vi "DeleteTempFolder.vi"(8 "error in (no error)":errorcluster, 10 "Project":string, 11 "Root":path) -> (0 "error out":errorcluster)   [LabVIEW 2019]
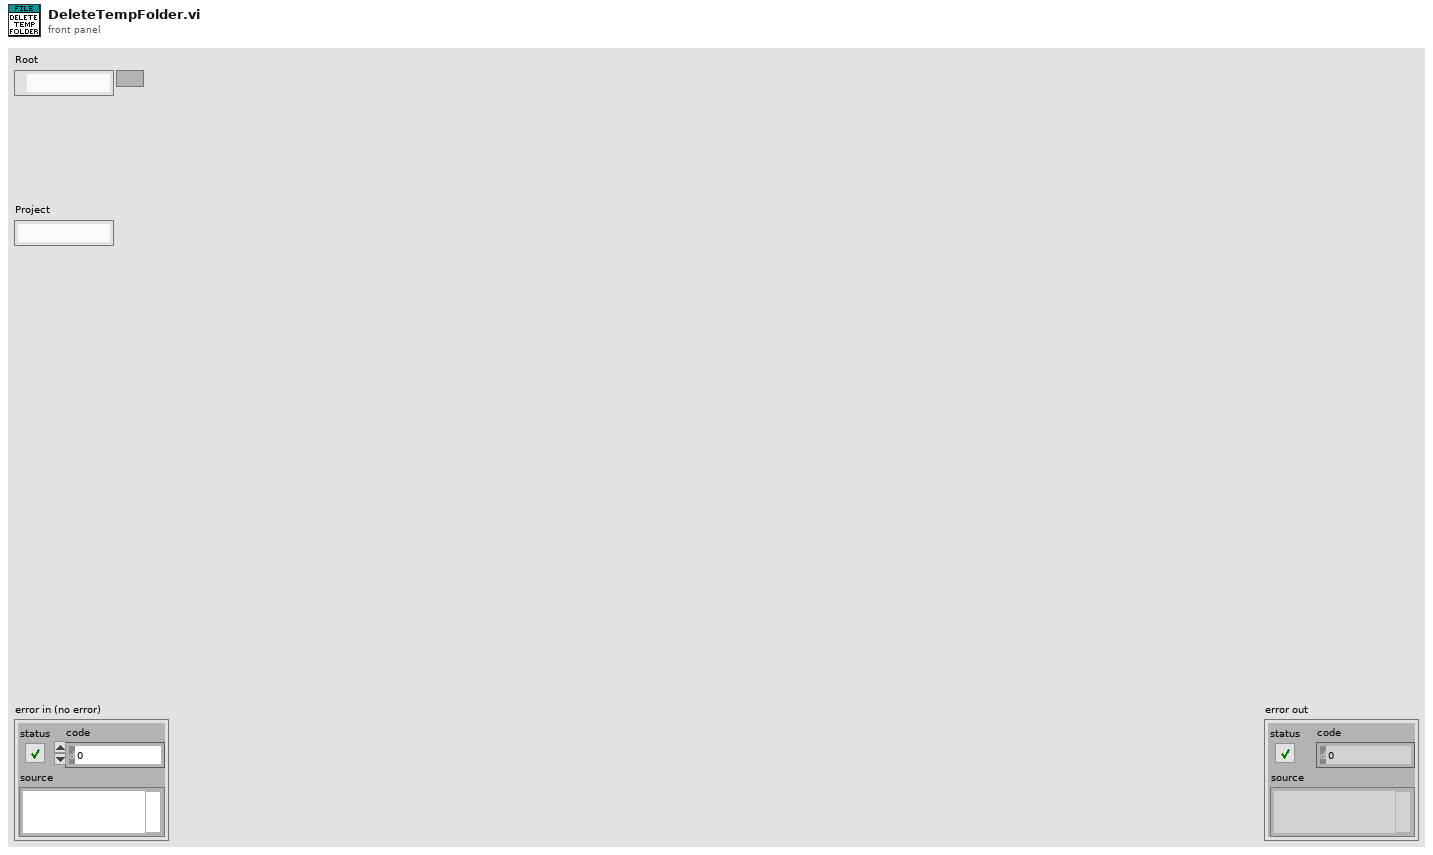
[diagram p1: front panel]
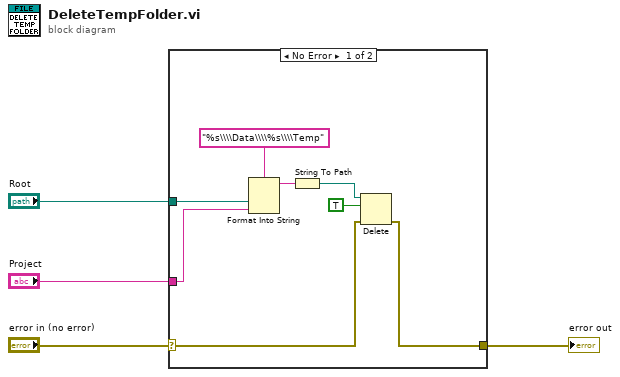
[diagram p0: block diagram]
diagram:
  n1 = case shown="No Error" "error in (no error)" {
    selector: "error in (no error)" -> [w6 w13]
    tunnel: "Root" -> [w12 _]
    tunnel: [w5 w13] -> w2
    tunnel: "Project" -> [w10 _]
    frame No Error {
      n2 = Format Into String(format string="%s\\\\Data\\\\%s\\\\Temp", w12, w10) -> (resulting string=w9:string)  [unwired: 2 in, 1 out]
      n3 = String To Path(string=w9) -> (path=w8:path)
      n4 = Delete(path (use dialog)=w8, entire hierarchy (F)=TRUE, error in=w6) -> (error out=w5:errorcluster)  [unwired: 2 in, 2 out]
    }
    frame Error {
    }
  }
  "error out" <- w2
